vi "Host-OrderBook-Deserialize-Results.vi"(11 "Data in":u64[](array[numeric])) -> (3 "OrderBook Array":T1(array[cluster]))   [LabVIEW 2016]
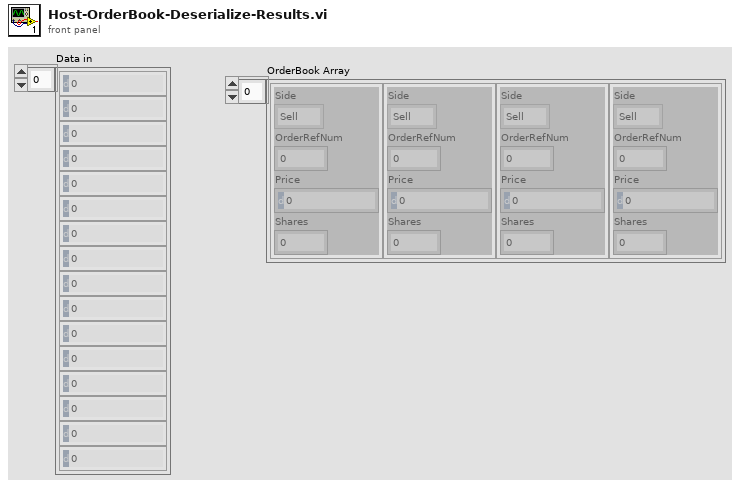
[diagram p1: front panel]
types:
  T1 = cluster{"Side":enum16{"Sell", "Buy"}, "OrderRefNum":u64, "Price":u32, "Shares":u32}[]
  T2 = cluster{"Side":enum16{"Sell", "Buy"}, "OrderRefNum":u64, "Price":u32, "Shares":u32}
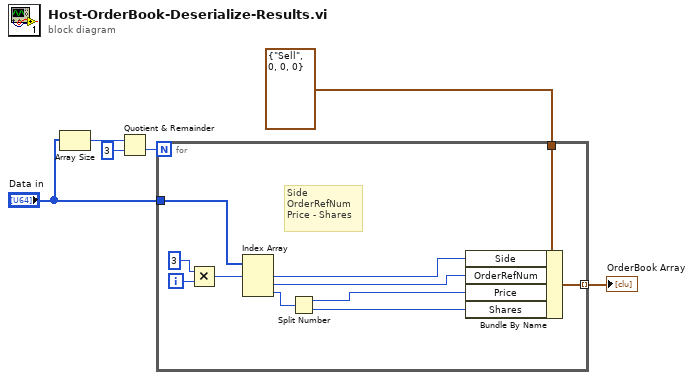
[diagram p0: block diagram]
diagram:
  n1 = Array Size(array="Data in") -> (size(s)=w6:i32)
  n2 = Quotient & Remainder(x=w6, y=3) -> (floor(x/y)=w4:i32)  [unwired: 1 out]
  n3 = for {
    N: w4 -> [_]
    tunnel: T2 {"Side"=enum."Sell", "OrderRefNum"=0, "Price"=0, "Shares"=0} ("Cluster") -> [w12]
    tunnel: [w13] -> w1 mode=indexing
    tunnel: "Data in" -> [w15]
    i -> [w17]
    # "Side\nOrderRefNum\nPrice - Shares"
    n4 = Multiply(x=3, y=w17) -> (x*y=w14:i32)
    n5 = Index Array(array=w15, index #1=w14) -> (element #1=w7:u64, element #2=w10:u64, element #3=w9:u64)  [unwired: 2 in]
    n6 = Split Number(x=w9) -> (hi(x)=w8:u32, lo(x)=w11:u32)
    n7 = Bundle By Name(cluster=w12, "Side"=w7, "OrderRefNum"=w10, "Price"=w8, "Shares"=w11) -> (w13:T2)
  }
  "OrderBook Array" <- w1
